vi "ex5 resolution d'une equation de 2eme degre.vi"() -> ()   [LabVIEW 2018]
panel:
  out "sc 2":csg
  out "sc1":csg
  out "s2":dbl
  out "s 1":dbl
  in  "c":dbl
  in  "b":dbl
  in  "a":dbl
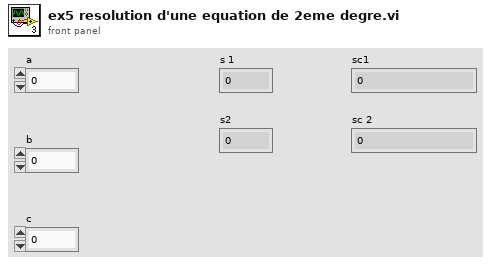
[diagram p1: front panel]
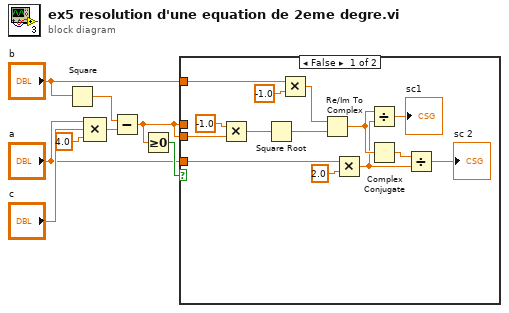
[diagram p0: block diagram]
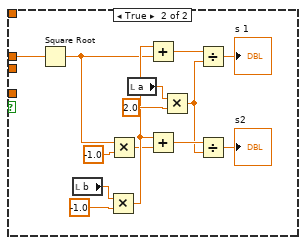
[diagram p2: hidden frame]
diagram:
  n1 = Square(x="b") -> (x^2=w6:dbl)
  n2 = Compound Arithmetic op=MULTIPLY("a", "c", 4.0 ("value")) -> (w5:dbl)
  n3 = Subtract(x=w6, y=w5) -> (x-y=w2:dbl)
  n4 = Greater Or Equal To 0?(x=w2) -> (x >= 0?=w4:bool)
  n5 = case shown="False" w4 {
    tunnel: w2 -> [_ w34]
    tunnel: "b" -> [w21 _]
    tunnel: w2 -> [w20 _]
    tunnel: "a" -> [w17 _]
    frame False {
      n6 = Multiply(x=-1.0, y=w20) -> (x*y=w18:dbl)
      n7 = Square Root(x=w18) -> (sqrt(x)=w15:dbl)
      n8 = Multiply(x=w21, y=-1.0) -> (x*y=w14:dbl)
      n9 = Re/Im To Complex(1:w15, 2:w14) -> (0:w12:cdb)
      n10 = Multiply(x=w17, y=2.0) -> (x*y=w10:dbl)
      n11 = Divide(x=w12, y=w10) -> (x/y=→"sc1":cdb)
      n12 = Complex Conjugate(1:w12) -> (0:w11:cdb)
      n13 = Divide(x=w11, y=w10) -> (x/y=→"sc 2":cdb)
    }
    frame True {
      n14 = Square Root(x=w34) -> (sqrt(x)=w28:dbl)
      n15 = local read "b"() -> (w36:dbl)
      n16 = Multiply(x=w36, y=-1.0) -> (x*y=w29:dbl)
      n17 = Multiply(x=w28, y=-1.0) -> (x*y=w26:dbl)
      n18 = local read "a"() -> (w33:dbl)
      n19 = Add(x=w29, y=w28) -> (x+y=w30:dbl)
      n20 = Add(x=w29, y=w26) -> (x+y=w25:dbl)
      n21 = Multiply(x=w33, y=2.0) -> (x*y=w24:dbl)
      n22 = Divide(x=w30, y=w24) -> (x/y=→"s 1":dbl)
      n23 = Divide(x=w25, y=w24) -> (x/y=→"s2":dbl)
    }
  }
